vi "Write Waveforms.vi"(8 "error in (no error)":errorcluster, 10 "Waveforms":waveform(dbl)[](array[waveform]), 11 "Abstract Fgen":refnum<class "Fgen Instrument.lvclass">) -> (0 "error out":errorcluster, 3 "Abstract Fgen out":refnum<class "Fgen Instrument.lvclass">)   [LabVIEW 2025]
uses:
  Fgen Instrument.lvclass
  Fgen Instrument.lvclass/Fgen Instrument.ctl
  C:/Users/Public/Documents/Sandia National Labs/TSS Plugin/Abstract Engine.lvlibp/Plugin/Abstract/Abstract Instrument/Abstract Instrument.lvclass
  C:/Users/Public/Documents/Sandia National Labs/TSS Plugin/CEF.lvlibp/serializable node/CEF_serializable node.lvclass
  C:/Users/Public/Documents/Sandia National Labs/TSS Plugin/CEF.lvlibp/Node/CEF_Node.lvclass
  C:/Working copy/tss/Plugin/Engines/Fgen/Fgen Instrument/Fgen Instrument.lvclass
  C:/Users/Public/Documents/Sandia National Labs/TSS Plugin/Interface.lvlibp/Analog Output/AO.lvclass
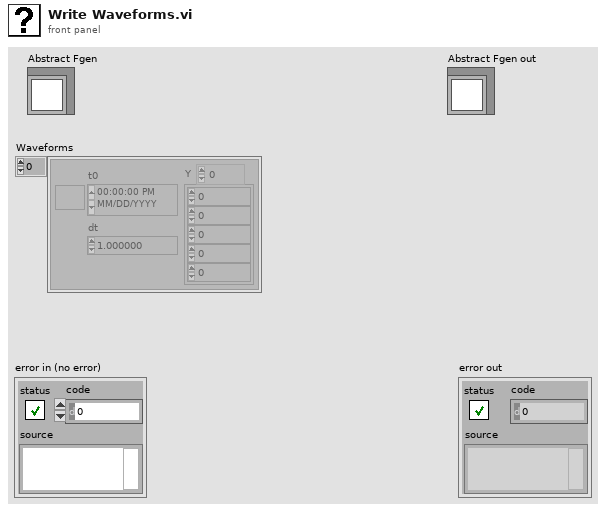
[diagram p1: front panel]
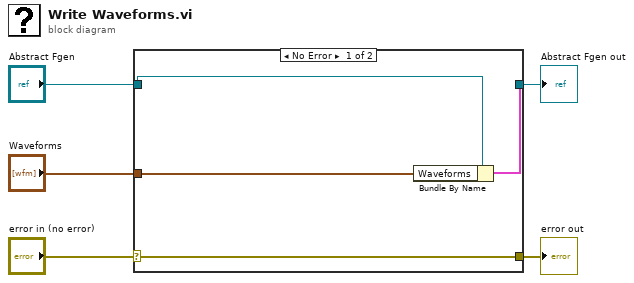
[diagram p0: block diagram]
diagram:
  n1 = case shown="No Error" "error in (no error)" {
    selector: "error in (no error)" -> [w9 w10]
    tunnel: [w9 w10] -> w4
    tunnel: [w7 w11] -> w1
    tunnel: "Abstract Fgen" -> [w8 w11]
    tunnel: "Waveforms" -> [w6 _]
    frame No Error {
      n2 = Bundle By Name(cluster=w8, "Waveforms"=w6) -> (w7:cluster{})
    }
    frame Error {
    }
  }
  "error out" <- w4
  "Abstract Fgen out" <- w1
